vi "Resampling for Simple DAQ.vi"(1 "Resample Index":u32[](array[numeric]), 2 "Points Per A-Scan":u32, 3 "U16 Array":u16[](array[numeric])) -> (0 "Array":u16[](array[numeric]))   [LabVIEW 2014]
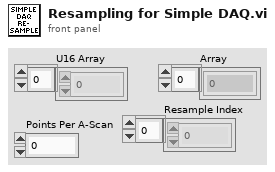
[diagram p1: front panel]
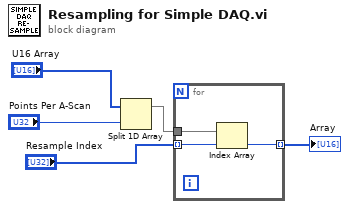
[diagram p0: block diagram]
diagram:
  n1 = Split 1D Array(array="U16 Array", index="Points Per A-Scan") -> (first subarray=w3:u16[])  [unwired: 1 out]
  n2 = for {
    tunnel: w3 -> [w8]
    tunnel: "Resample Index" -> [w7] mode=indexing
    tunnel: [w6] -> w1 mode=indexing
    n3 = Index Array(array=w8, index=w7) -> (element=w6:u16)
  }
  "Array" <- w1
